vi "SMO.UI.ErrorTester.GenerateError.vi"(8 "error in (no error)":errorcluster, 10 "code":i32, 11 "SMO.UI.ByRefWithEvents":refnum<class "SMO.UI.ErrorTester.lvclass">) -> (0 "error out":errorcluster, 3 "SMO.UI.ByRefWithEvents out":refnum<class "SMO.UI.ErrorTester.lvclass">)   [LabVIEW 2013, in "SMO.UI.ErrorTester.lvclass"]
doc: "---------------------------------------------------------------\nJKI State Machine Objects™\nhttp://jki.net/state-machine-objects/\nCopyright (C) 2005-2015, JKI <info@jki.net>\nALL RIGHTS RESERVEDJKI State Machine Objects (SMO) 1.0.0.5\nJKI - JKI\nCopyright (c) 2016, JKI"
uses:
  SMO.UI.ErrorTester.lvclass
  Typedefs/GenerateError--Cluster.ctl
panel:
  # "For instructions on how to use the JKI State Machine Objects, examples and video tutorials, visit:\nhttp://jki.net/state-machine-objects/\n\nJKI State Machine Objects™\nhttp://jki.net/state-machine-objects/\nCopyright (C) 2005-2015, JKI <info@jki.net>\nALL RIGHTS RESERVED"
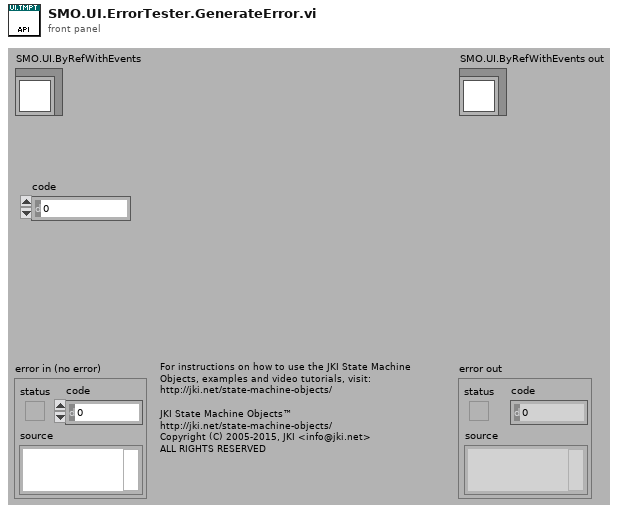
[diagram p1: front panel]
types:
  T1 = typedef "SMO.UI.ErrorTester.lvclass/GenerateError--Cluster.ctl" = cluster{"error":errorcluster}
  T2 = typedef "SMO.UI.ErrorTester.lvclass/ProtectedEvents--Cluster.ctl" = cluster{"ErrorGeneration":refnum<user-event>}
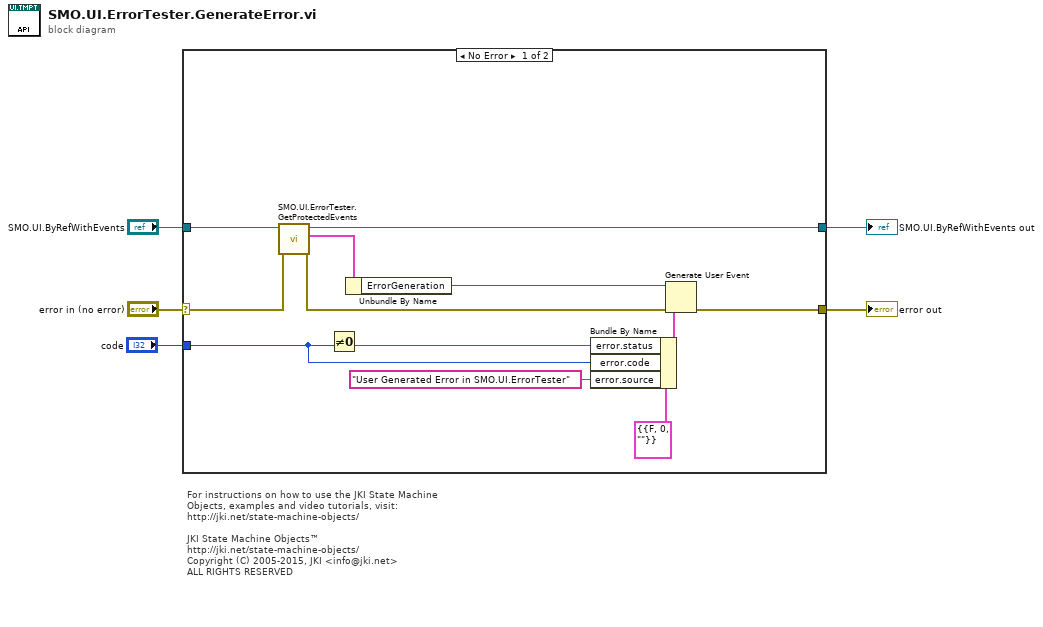
[diagram p0: block diagram]
diagram:
  # "For instructions on how to use the JKI State Machine Objects, examples and video tutorials, visit:\nhttp://jki.net/state-machine-objects/\n\nJKI State Machine Objects™\nhttp://jki.net/state-machine-objects/\nCopyright (C) 2005-2015, JKI <info@jki.net>\nALL RIGHTS RESERVED"
  n1 = case shown="No Error" "error in (no error)" {
    selector: "error in (no error)" -> [w17 w18]
    tunnel: "SMO.UI.ByRefWithEvents" -> [w14 w19]
    tunnel: [w16 w18] -> w4
    tunnel: [w15 w19] -> w3
    tunnel: "code" -> [w7 _]
    frame No Error {
      n2 = call "SMO.UI.ErrorTester.GetProtectedEvents.vi"("error in (no error)"=w17, "SMO.UI.ByRefWithEvents"=w14) -> ("error out"=w11:errorcluster, "Protected Events"=w12:T2, "SMO.UI.ByRefWithEvents out"=w15:refnum<class "SMO.UI.ErrorTester.lvclass">)  [unwired: 7 in]
      n3 = Not Equal To 0?(x=w7) -> (x != 0?=w8:bool)
      n4 = Unbundle By Name(w12) -> ("ErrorGeneration"=w13:refnum<user-event>)
      n5 = Bundle By Name(cluster=T1 {"error"={"status"=FALSE, "code"=0, "source"=""}} ("event data"), "error.status"=w8, "error.code"=w7, "error.source"="User Generated Error in SMO.UI.ErrorTester") -> (w9:T1)
      n6 = Generate User Event(user event=w13, event data cluster=w9, error in=w11) -> (error out=w16:errorcluster)  [unwired: 1 in, 1 out]
    }
    frame Error {
    }
  }
  "error out" <- w4
  "SMO.UI.ByRefWithEvents out" <- w3
